vi "ProjectRun.vi"(8 "error in (no error)":errorcluster) -> (0 "error out":errorcluster)   [LabVIEW 2015, in "ni-veristand-steps-runtime-lib.lvlib"]
uses:
  ni-veristand-steps-runtime-lib.lvlib
  <vilib>/NI Veristand/Execution/Project/NI_VS Project ExecutionAPI.lvlib
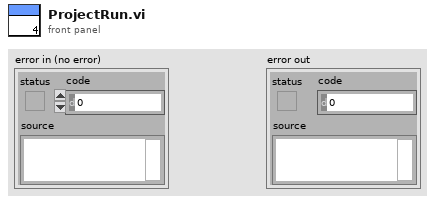
[diagram p1: front panel]
types:
  T1 = typedef "ni-veristand-steps-runtime-lib.lvlib/VeriStand dotNet References.ctl" = cluster{"Project Ref":refnum<k24>, "Workspace Manager Ref":refnum<k24>, "Model Manager Ref":refnum<k24>, "Channel Fault Manager Ref":refnum<k24>}
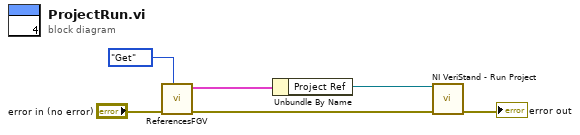
[diagram p0: block diagram]
diagram:
  n1 = call "ReferencesFGV.vi"("Get/Set"=enum16{"Get", "Set"}."Get", "error in (no error)"="error in (no error)") -> ("error out"=w2:errorcluster, "VeriStand dotNET Refs out"=w5:T1)  [unwired: 8 in]
  n2 = Unbundle By Name(w5) -> ("Project Ref"=w1:refnum<k24>)
  n3 = call <vilib>:"NI VeriStand - Run Project.vi"("error in (no error)"=w2, "Project Ref in"=w1) -> ("error out"=→"error out":errorcluster)  [unwired: 8 in, 1 out]
